vi "System_PXIe.vi"() -> ()   [LabVIEW 2017]
panel:
  out "Core Closing Error":errorcluster
  out "VFD Closing Error":errorcluster
  out "DAQ Closing Error":errorcluster
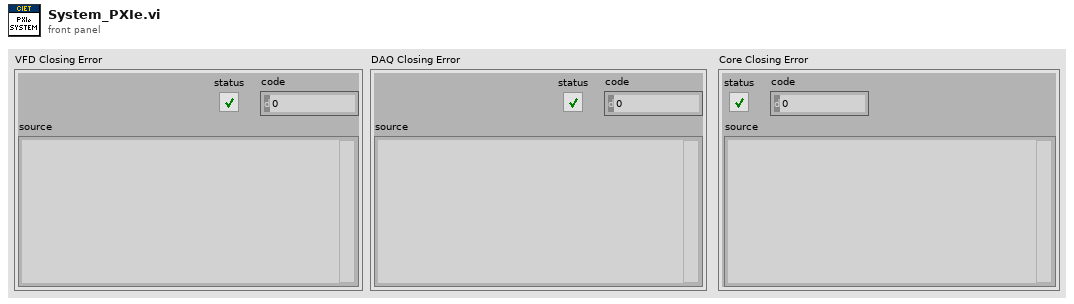
[diagram p1: front panel]
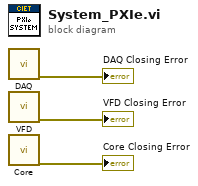
[diagram p0: block diagram]
diagram:
  n1 = call "DAQ.vi"() -> ("Error Out"=→"DAQ Closing Error":errorcluster)  [unwired: 11 in]
  n2 = call "VFD.vi"() -> ("GS1 Communication Error Out"=→"VFD Closing Error":errorcluster)  [unwired: 11 in]
  n3 = call "Core.vi"() -> ("Error Out"=→"Core Closing Error":errorcluster)  [unwired: 19 in]
